vi "StringToI16(cast).vi"(1 "String":string) -> (0 "I16":i16)   [LabVIEW 2012]
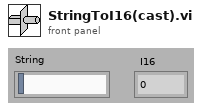
[diagram p1: front panel]
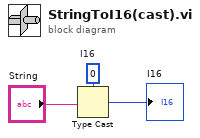
[diagram p0: block diagram]
diagram:
  w2 = i16 0  # I16
  n1 = Type Cast(type=w2, x="String") -> (*(type *) &x=→"I16":i16)
